vi "DG535.set trigger mode.vi"(0 "i ref in":refnum<vi>, 7 "Trigger Mode":i32(ring) items=["Internal", "External", "Single Shot", "Burst"], 11 "error in":errorcluster) -> (4 "i ref out":refnum<vi>, 15 "error out":errorcluster)   [LabVIEW 2014, in "DG535.lvlib"]
uses:
  DG535.lvlib
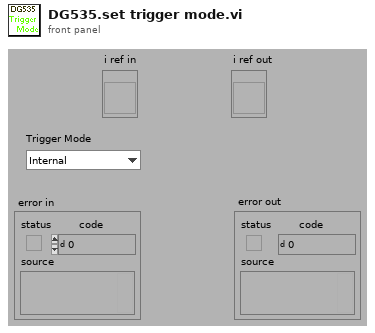
[diagram p1: front panel]
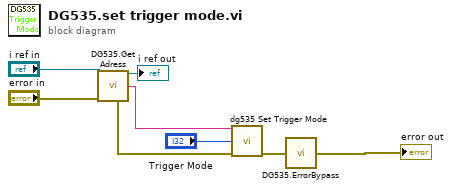
[diagram p0: block diagram]
diagram:
  n1 = call "DG535.Get Adress.vi"("i ref in"="i ref in", "error in (no error)"="error in") -> ("i ref out"=→"i ref out":refnum<vi>, "address"=w6:string, "error out"=w5:errorcluster)  [unwired: 10 in, 1 out]
  n2 = call "dg535 Set Trigger Mode.vi"("address string"=w6, "Trigger Mode"="Trigger Mode", "error in"=w5) -> ("error out"=w7:errorcluster)  [unwired: 12 in]
  n3 = call "DG535.ErrorBypass.vi"("error in (no error)"=w7) -> ("error out"=→"error out":errorcluster)  [unwired: 14 in]
